vi "Init Actor Core.vi"(8 "error in (no error)":errorcluster, 11 "Measure Object in":refnum<class "Measure Object.lvclass">) -> (0 "error out":errorcluster, 3 "Measure Object out":refnum<class "Measure Object.lvclass">)   [LabVIEW 2015, in "Measure Object.lvclass"]
uses:
  Measure Object.lvclass
  Measure Object.lvclass/Measure Object.ctl
  Read Name.vi
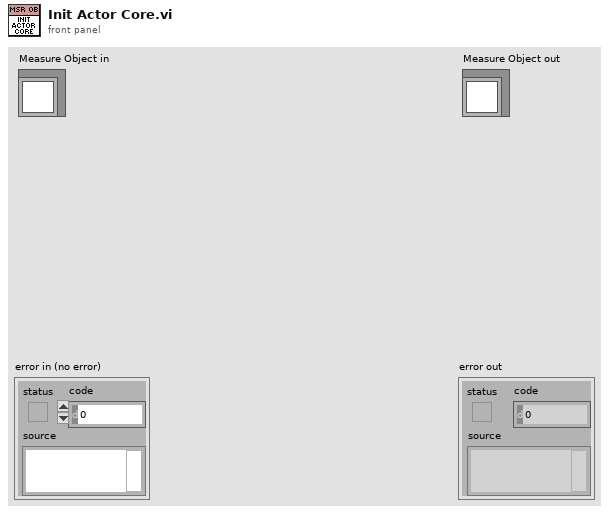
[diagram p1: front panel]
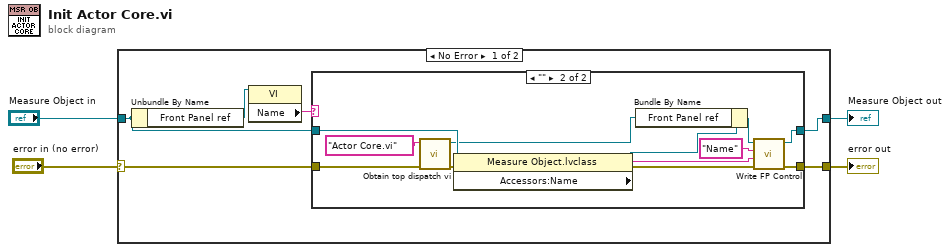
[diagram p0: block diagram]
diagram:
  n1 = case shown="No Error" "error in (no error)" {
    selector: "error in (no error)" -> [w8 w26]
    tunnel: [w7 w26] -> w3
    tunnel: [w5 w25] -> w1
    tunnel: "Measure Object in" -> [w6 w25]
    frame No Error {
      n2 = Unbundle By Name(w6) -> ("Front Panel ref"=w10:refnum<vi>)
      n3 = property class="VI"(reference=w10) -> ("Name"=w9:string)  [unwired: 1 in, 2 out]
      n4 = case shown="\"\"" w9 {
        tunnel: w8 -> [w12 w23]
        tunnel: w6 -> [w11 w22]
        tunnel: [w12 w18] -> w7
        tunnel: [w11 w19] -> w5
        frame Default {
        }
        frame "" {
          n5 = call "Obtain top dispatch vi.vi"("Error In"=w23, "VI name"="Actor Core.vi") -> ("Error Out"=w14:errorcluster, "vi reference"=w21:refnum<vi>)  [unwired: 7 in, 1 out]
          n6 = property class="Measure Object.lvclass"(reference=w22, error in=w14) -> (reference out=w16:refnum<class "Measure Object.lvclass">, error out=w13:errorcluster, "Accessors:Name"=w15:string)
          n7 = Bundle By Name(cluster=w16, "Front Panel ref"=w21) -> (w20:refnum<class "Measure Object.lvclass">)
          n8 = call-dynamic "Write FP Control.vi"("error in (no error)"=w13, "Control Value"=w15, "Control Name"="Name", "Measure Object in"=w20) -> ("error out"=w18:errorcluster, "Measure Object out"=w19:refnum<class "Measure Object.lvclass">)  [unwired: 6 in]
        }
      }
    }
    frame Error {
    }
  }
  "error out" <- w3
  "Measure Object out" <- w1
